vi "Get Last Path Segment.vi"(11 "String in":string) -> (3 "String out":string)   [LabVIEW 2017]
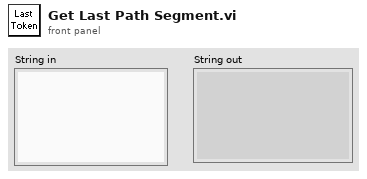
[diagram p1: front panel]
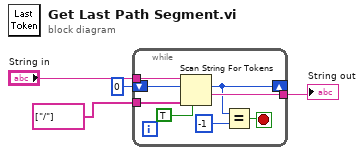
[diagram p0: block diagram]
diagram:
  n1 = while {
    tunnel: "String in" -> [w12]
    tunnel: string[] ["/"] ("delimiters (\\s,\\t,\\r,\\n)") -> [w11]
    shift-right: [w7] -> _
    shift-left: 0 ("offset past token") -> [w10]
    tunnel: [w8] -> w2
    stop <- w5 stop-if-true
    n2 = Scan String For Tokens(4:TRUE ("use cached delim/oper data? (F)"), 6:w11, 8:w10, 9:w12) -> (1:w8:string, 2:w7:i32)  [unwired: 2 in, 2 out]
    n3 = Equal?(x=w7, y=-1) -> (x = y?=w5:bool)
  }
  "String out" <- w2
